vi "Lian_Lab01_I.vi"() -> ()   [LabVIEW 2020]
uses:
  <vilib>/Analysis/NI_AALBase.lvlib
  <vilib>/measure/NI_MABase.lvlib
panel:
  in  "Frequency":dbl=10.0 format="%0.2p"
  in  "Offset":dbl format="%0.2p"
  in  "Samples":i32=128
  in  "Sampling Info":cluster{"Fs":dbl, "#s":dbl}={"Fs"=1000.0, "#s"=1000.0} {"Fs" format="%.2p"}
  in  "Phase":dbl
  in  "Offset":dbl
  in  "Amplitude":dbl
  in  "Frequency":dbl
  out "Waveform Graph 3":dynamicdata(graph)
  in  "Phase":dbl
  in  "Amplitude":dbl
  out "Waveform Graph 2":waveform(dbl)(graph)
  in  "Phase In":dbl
  in  "Amplitude":dbl
  in  "Frequency":dbl
  out "Waveform Graph 1":dbl[](graph)
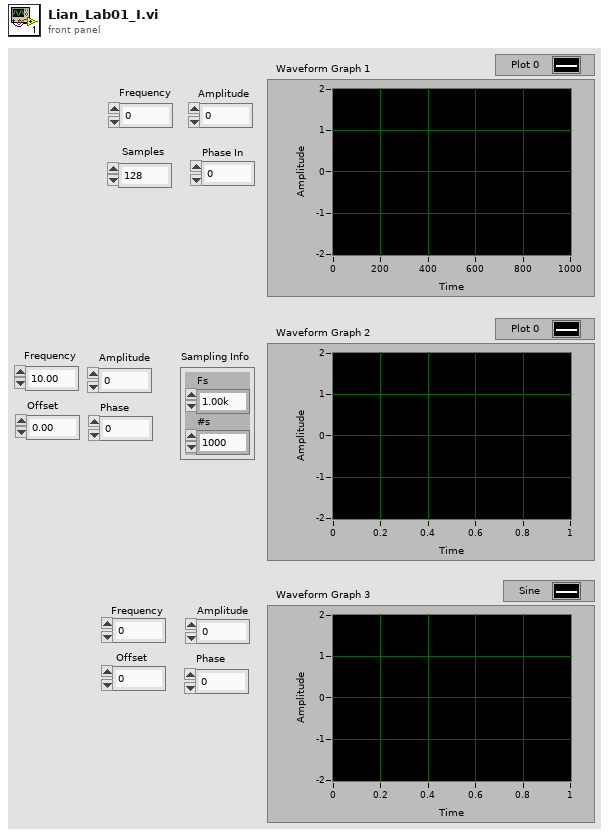
[diagram p1: front panel]
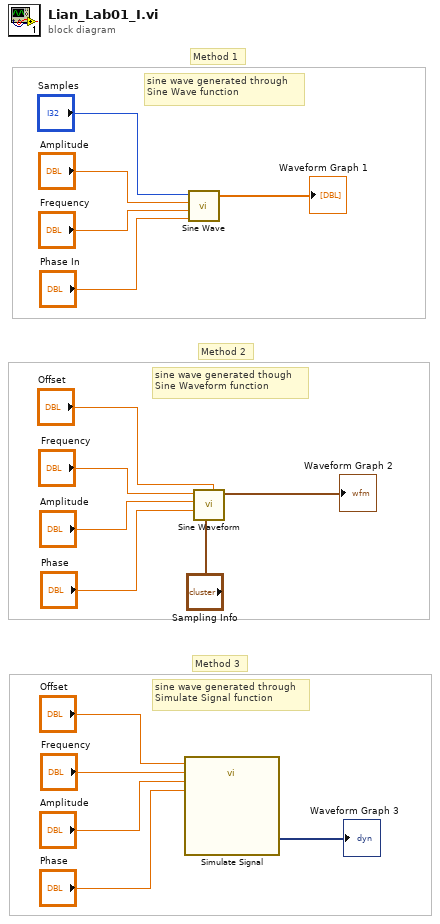
[diagram p0: block diagram]
diagram:
  # "Method 3"
  # "Method 2"
  # "Method 1"
  # "sine wave generated through\nSimulate Signal function"
  # "sine wave generated though \nSine Waveform function"
  # "sine wave generated through \nSine Wave function"
  n1 = call "Simulate Signal"("Offset"="Offset", "Frequency"="Frequency", "Amplitude"="Amplitude", "Phase"="Phase") -> ("Sine"=→"Waveform Graph 3":dynamicdata)  [unwired: 10 in, 1 out]
  n2 = call <vilib>:"Sine Wave.vi"("samples"="Samples", "amplitude"="Amplitude", "frequency"="Frequency", "phase in"="Phase In") -> ("sine wave"=→"Waveform Graph 1":dbl[])  [unwired: 1 in, 2 out]
  n3 = call <vilib>:"Sine Waveform.vi"("offset"="Offset", "sampling info"="Sampling Info", "phase"="Phase", "amplitude"="Amplitude", "frequency"="Frequency") -> ("signal out"=→"Waveform Graph 2":waveform(dbl))  [unwired: 5 in, 1 out]
